vi "Process.vi"(8 "error in":errorcluster, 11 "RemoteControl":refnum<class "RemoteControl.lvclass">) -> (0 "error out":errorcluster, 3 "RemoteControl out":refnum<class "RemoteControl.lvclass">)   [LabVIEW 2020, in "RemoteControl.lvclass"]
doc: "---------------------------------------------------------------\nJKI State Machine Objects™\nhttp://jki.net/state-machine-objects/\nCopyright (C) 2005-2015, JKI <info@jki.net>\nALL RIGHTS RESERVED"
uses:
  RemoteControl.lvclass
  C:/Program Files (x86)/National Instruments/LabVIEW 2020/vi.lib/JKI/JKI SMO/SMO/SMO.lvclass
  Typedefs/RC Process Type--Enum.ctl
  Typedefs/Message--Cluster.ctl
  <vilib>/JKI/JKI SMO/SMO/Typedefs/Parent Call--Enum.ctl
  RemoteControl.lvclass/RemoteControl.ctl
  Typedefs/PublicEvents--RemoteControl.SendMessageFromProcess.ctl
  <vilib>/JKI/JKI SMO/SMO/Typedefs/SMOState --Enum.ctl
  LevyLab/LevyLab.lvclass
  <vilib>/JKI/JKI SMO/SMO/SMO.lvclass
panel:
  in  "Message Timing?":bool
  in  "timeout in ms (100)":i32=10
  out "Message from Remote":T1 {"Message ID" format="%#_6f"}
  out "Message from Owner":T1 {"Message ID" format="%#_6f"}
  in  "stop":bool
  out "RC Process Type":T2=enum."Server"
  # "For instructions on how to use the JKI State Machine Objects, examples and video tutorials, visit:\nhttp://jki.net/state-machine-objects/\n\nJKI State Machine Objects™\nhttp://jki.net/state-machine-objects/\nCopyright (C) 2005-2015, JKI <info@jki.net>\nALL RIGHTS RESERVED"
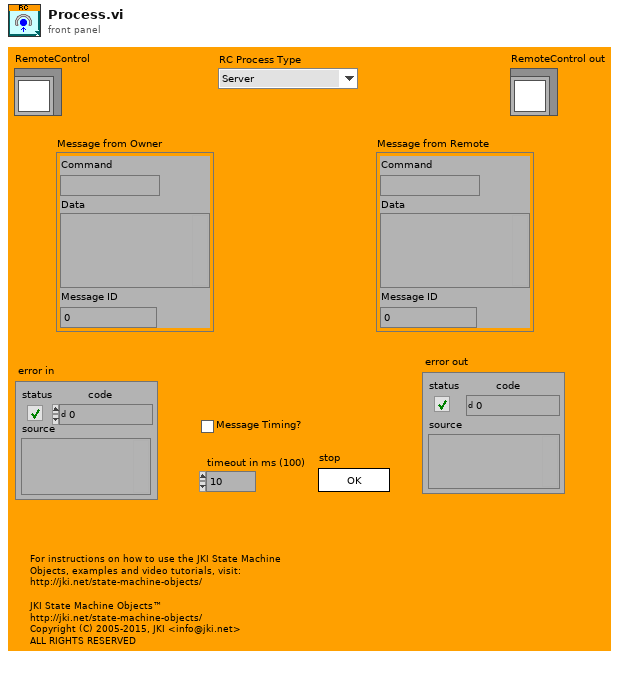
[diagram p1: front panel]
types:
  T1 = typedef "RemoteControl.lvclass/Message--Cluster.ctl" = cluster{"Command":string, "Data":variant, "Message ID":i32}
  T2 = typedef "RemoteControl.lvclass/RC Process Type--Enum.ctl" = enum16{"Connection Monitor", "Server", "Client"}
  T3 = typedef "SMO.lvclass/Parent Call--Enum.ctl" = enum16{"Allows parent to run", "Does not request parent to run"}
  T4 = enum32{"invalid app kind", "Development System", "Run Time System", "Student Edition", "Embedded LabVIEW", "Evaluation", "Custom"}
  T5 = enum32{"Invalid", "Standard", "Closed", "Hidden", "Minimized", "Maximized"}
  T6 = enum32{"Bad", "Idle", "Run top level", "Running"}
  T7 = typedef "RemoteControl.lvclass/PrivateEvents--RemoteControl.Configure.ctl" = cluster{"address":string, "Port":u16, "AllowedRemote":string, "Commands":string[], "Debug Mode?":bool}
  T8 = cluster{"Core":cluster{"Current VI Reference":refnum<vi>, "Close Panel on Exit?":bool, "error":errorcluster}, "Self Reference":refnum<class "RemoteControl.lvclass">, "RC Process Type":T2, "Configure":T7, "Message":T1, "Server":refnum<class "RemoteControl.lvclass">, "Debug Mode?":bool}
  T9 = cluster{"Current VI Reference":refnum<vi>, "Close Panel on Exit?":bool, "error":errorcluster}
  T10 = typedef "SMO.lvclass/Protected Events.ctl" = cluster{"StopProcesses":refnum<user-event>, "AbortProcesses":refnum<user-event>, "Config Changed":refnum<user-event>, "Dependency":refnum<user-event>}
  T11 = typedef "RemoteControl.lvclass/PrivateEvents--Cluster.ctl" = cluster{"Configure":refnum<user-event>, "SendMessageToProcess":refnum<user-event>}
  T12 = typedef "RemoteControl.lvclass/PublicEvents--Cluster.ctl" = cluster{"SendMessageFromProcess":refnum<user-event>}
  T13 = typedef "SMO.lvclass/Public Events.ctl" = cluster{"Error":refnum<user-event>, "State":refnum<user-event>, "Reserve State":refnum<user-event>}
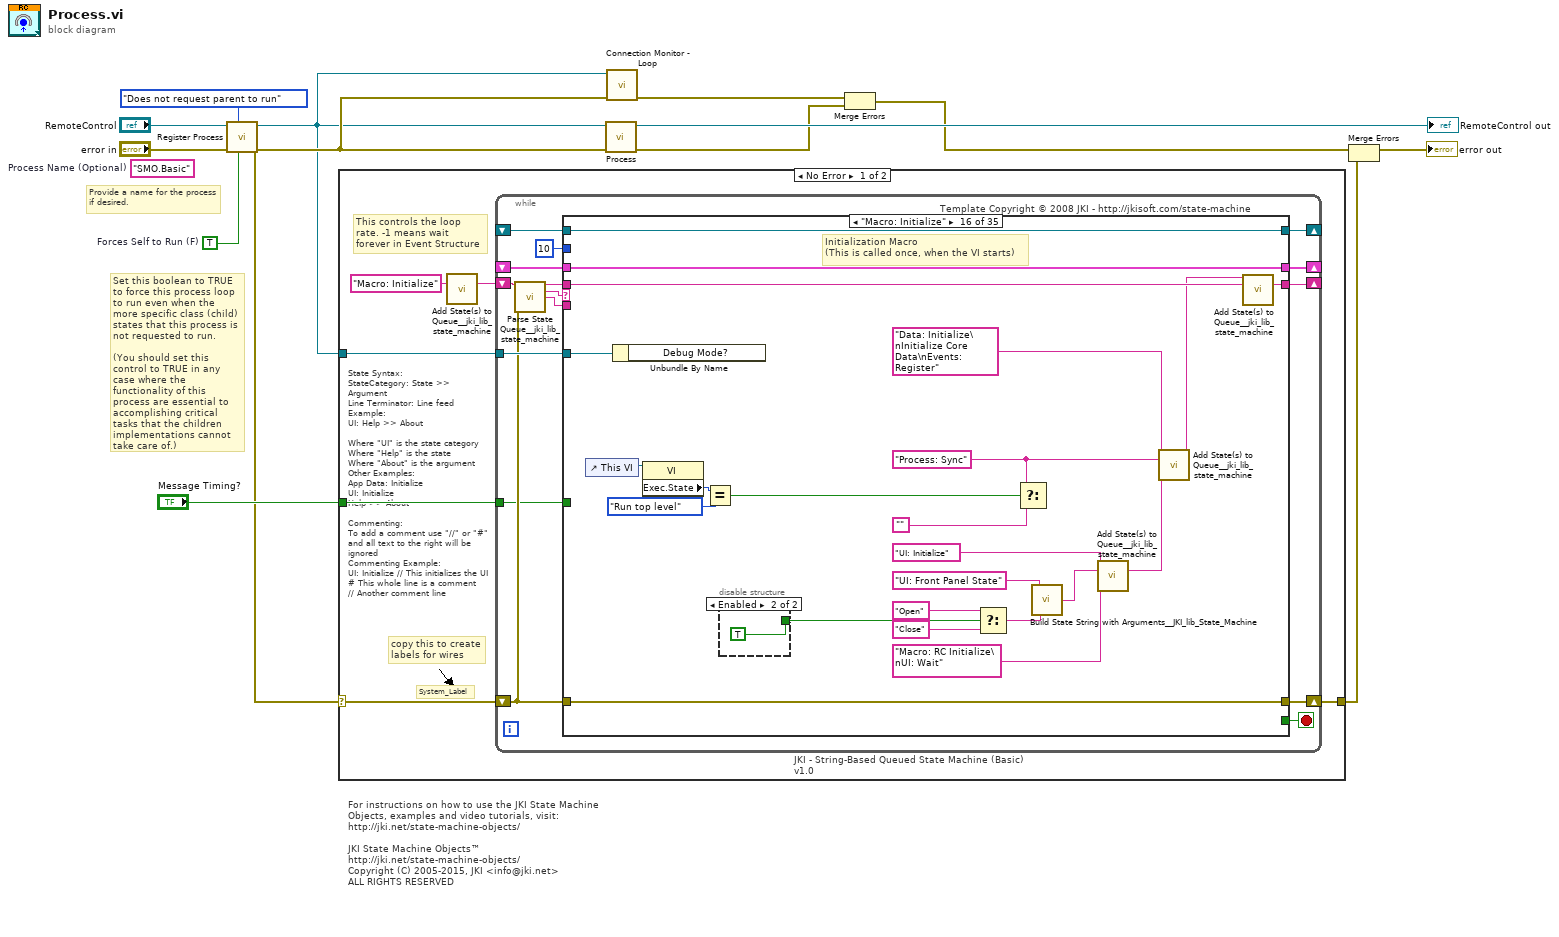
[diagram p0: block diagram]
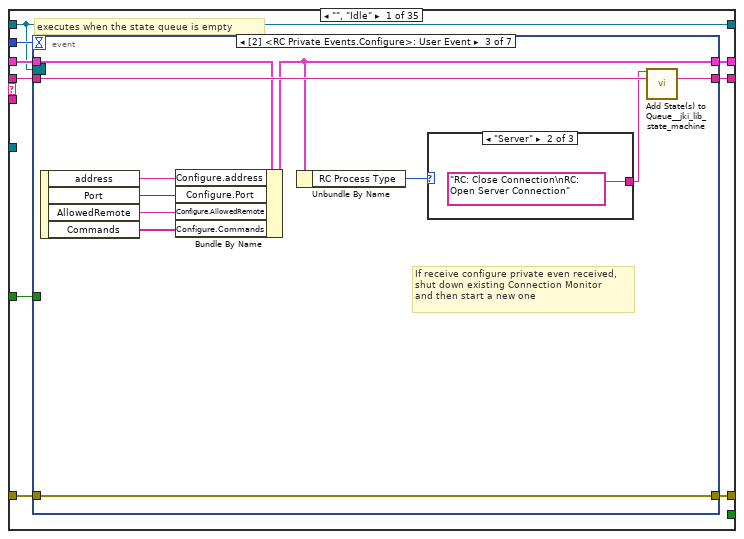
[diagram p2: hidden frame]
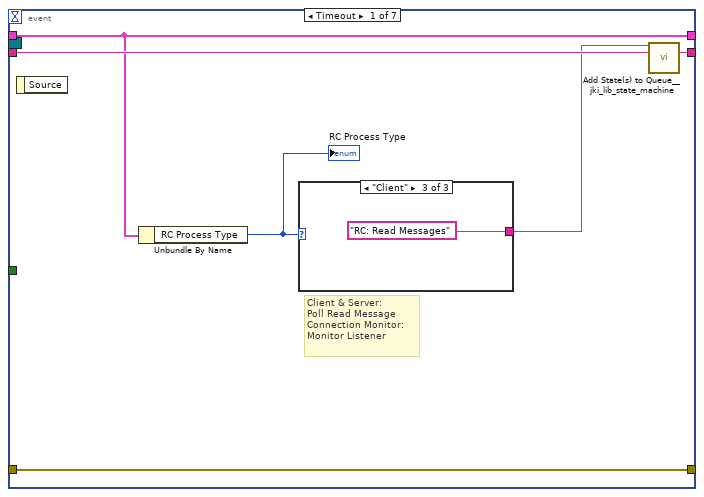
[diagram p3: hidden frame]
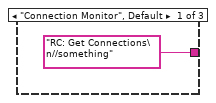
[diagram p4: hidden frame]
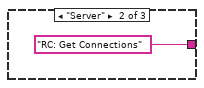
[diagram p5: hidden frame]
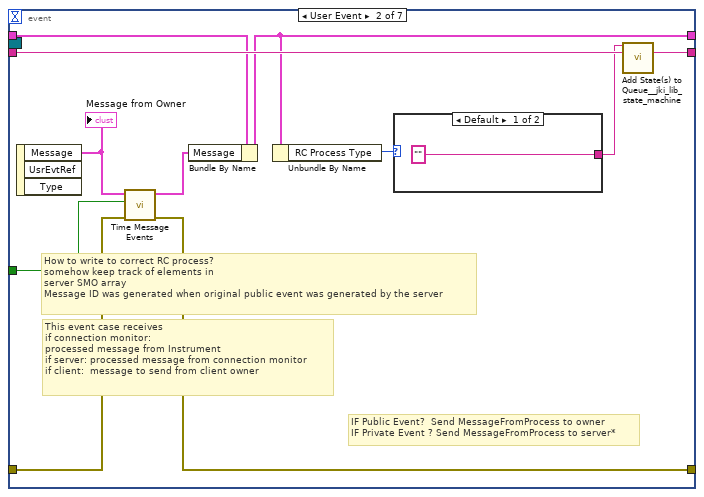
[diagram p6: hidden frame]
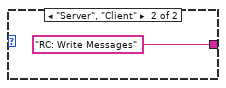
[diagram p7: hidden frame]
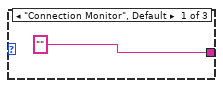
[diagram p8: hidden frame]
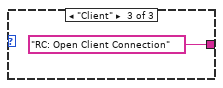
[diagram p9: hidden frame]
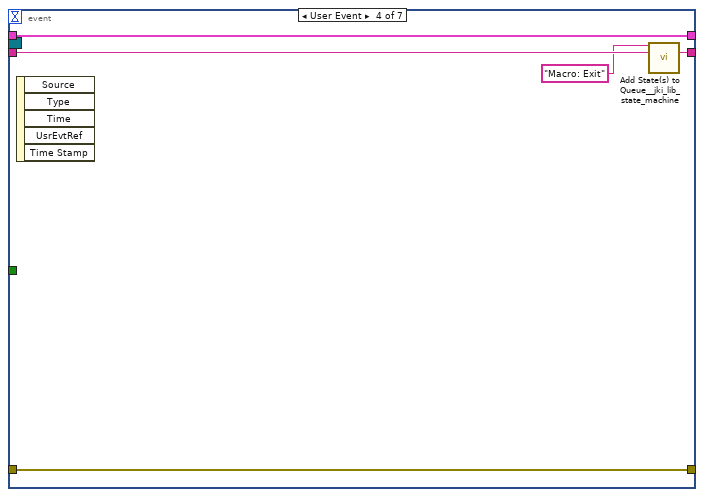
[diagram p10: hidden frame]
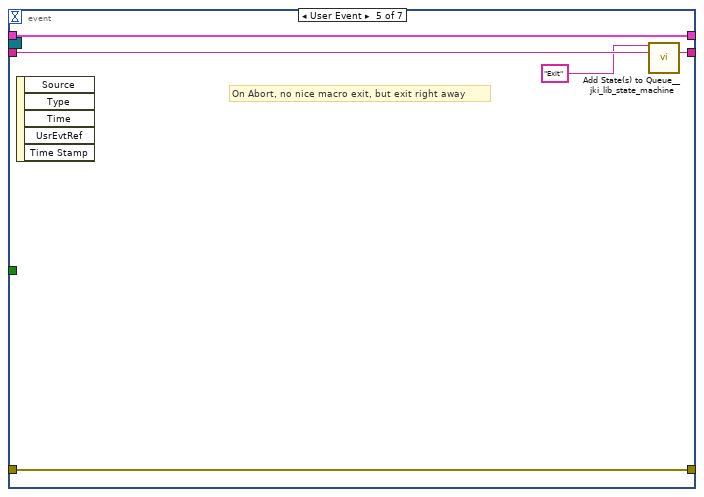
[diagram p11: hidden frame]
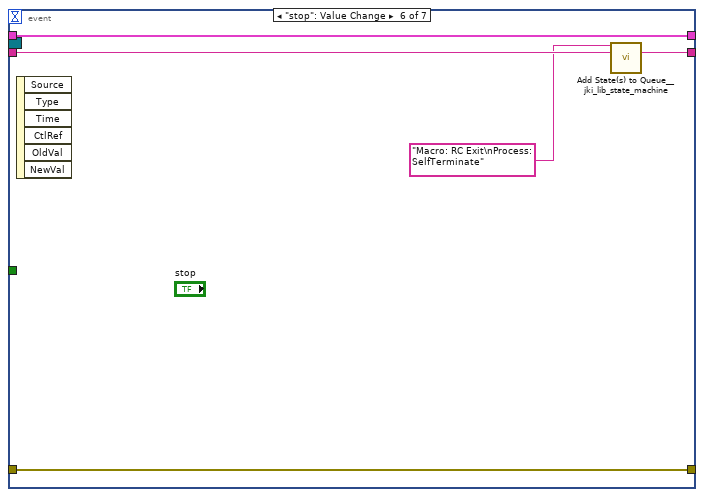
[diagram p12: hidden frame]
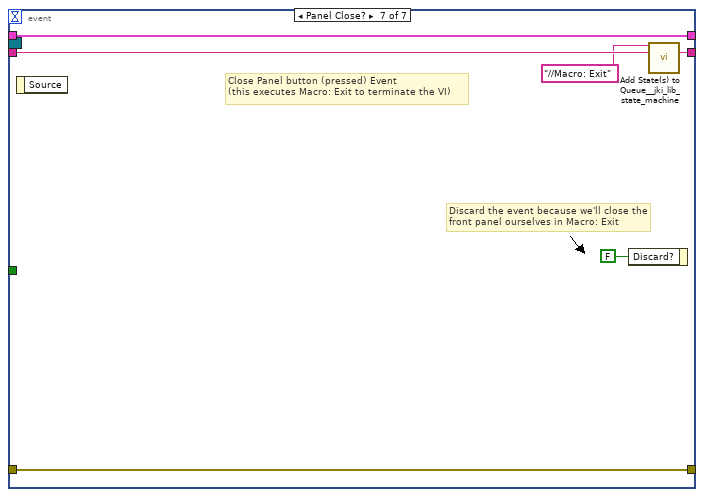
[diagram p13: hidden frame]
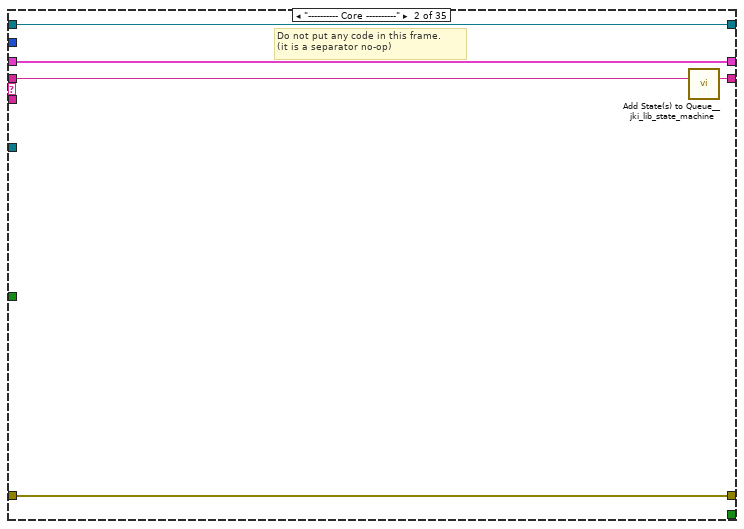
[diagram p14: hidden frame]
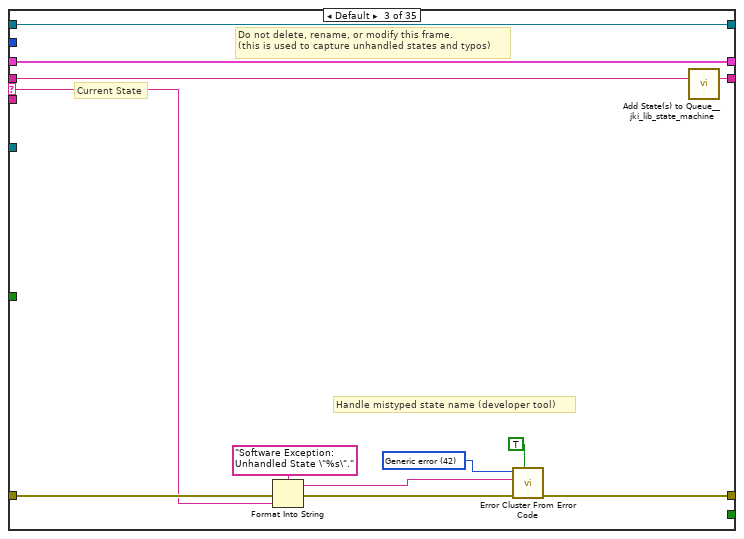
[diagram p15: hidden frame]
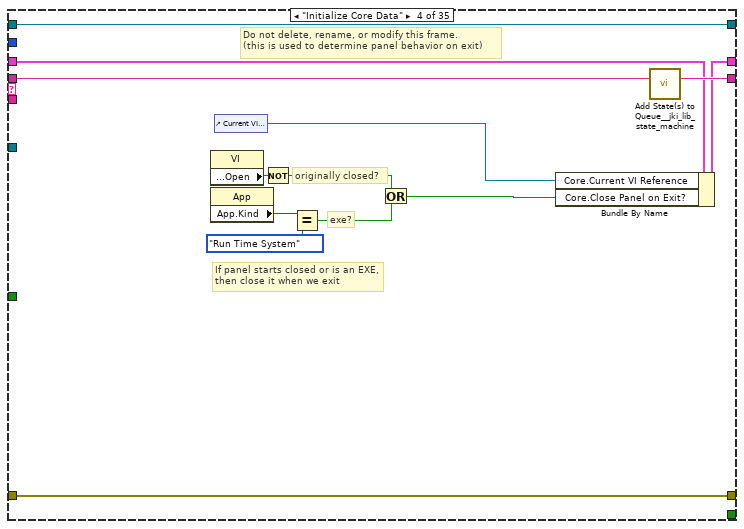
[diagram p16: hidden frame]
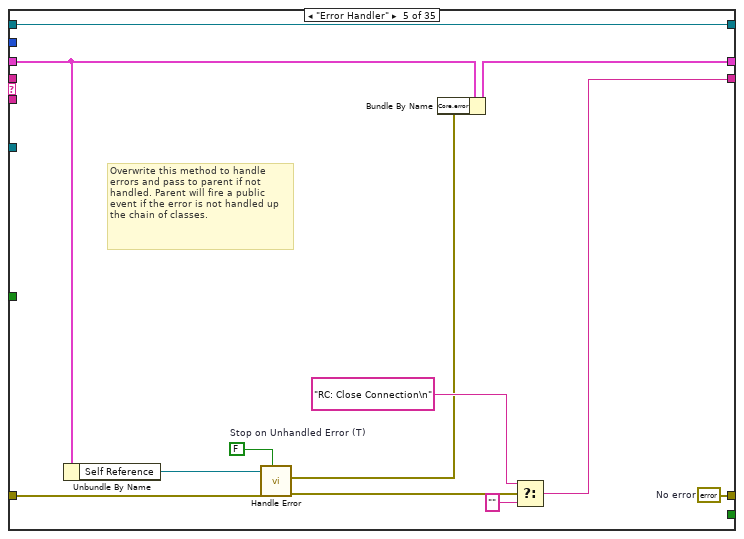
[diagram p17: hidden frame]
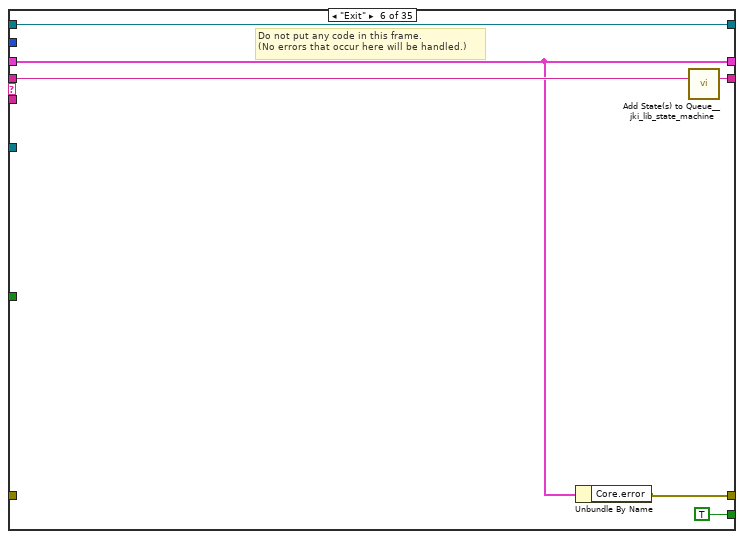
[diagram p18: hidden frame]
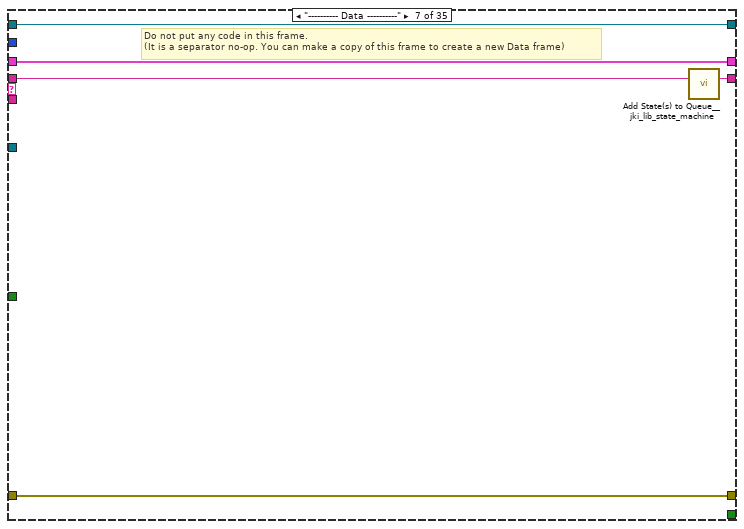
[diagram p19: hidden frame]
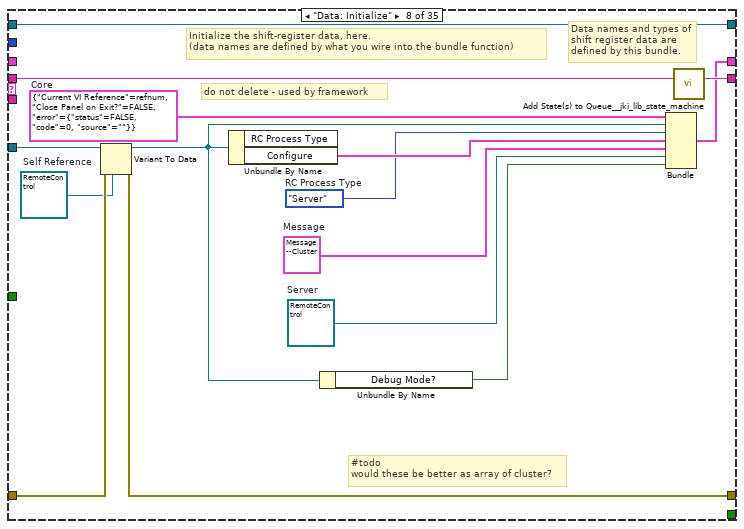
[diagram p20: hidden frame]
diagram:
  w7 = TRUE  # Forces Self to Run (F)
  (unwired) "SMO.Basic"  # Process Name (Optional)
  # "Provide a name for the process\nif desired."
  # "Set this boolean to TRUE to force this process loop to run even when the more specific class (child) states that this process is not requested to run.\n\n(You should set this control to TRUE in any case where the functionality of this process are essential to accomplishing critical tasks that the children implementations cannot take care of.)"
  # "For instructions on how to use the JKI State Machine Objects, examples and video tutorials, visit:\nhttp://jki.net/state-machine-objects/\n\nJKI State Machine Objects™\nhttp://jki.net/state-machine-objects/\nCopyright (C) 2005-2015, JKI <info@jki.net>\nALL RIGHTS RESERVED"
  n1 = call <vilib>:"Register Process.vi"("Forces Self to Run (F)"=w7, "Parent Call"=Parent_Call--Enum."Does not request parent to run", "error in (no error)"="error in", "SMO"="RemoteControl") -> ("error out"=w2:errorcluster, "SMO out"=w1:refnum<class "RemoteControl.lvclass">)  [unwired: 6 in]
  n2 = case shown="No Error" w2 {
    selector: w2 -> [w16 w489]
    tunnel: w1 -> [w17 _]
    tunnel: [w15 w489] -> w9
    tunnel: "Message Timing?" -> [w14 _]
    frame No Error {
      # "State Syntax:\nStateCategory: State >> Argument\nLine Terminator: Line feed\nExample:\nUI: Help >> About\n\nWhere \"UI\" is the state category\nWhere \"Help\" is the state\nWhere \"About\" is the argument\nOther Examples:\nApp Data: Initialize\nUI: Initialize\nHelp >> About\n\nCommenting:\nTo add a comment use \"//\" or \"#\" and all text to the right will be ignored\nCommenting Example:\nUI: Initialize // This initializes the UI\n# This whole line is a comment\n// Another comment line"
      # "copy this to create labels for wires"
      # "This controls the loop rate. -1 means wait forever in Event Structure"
      # "System_Label"
      n3 = call <vilib>:"Add State(s) to Queue__jki_lib_state_machine.vi"("State(s) in (\"\")"="Macro: Initialize") -> ("States Out"=w19:string)  [unwired: 14 in]
      n4 = while "JKI - String-Based Queued State Machine (Basic) v1.0" {
        shift-right: [w27] -> _
        shift-left: _ -> [w20]
        shift-right: [w30] -> w15
        shift-left: w16 -> [w22]
        shift-right: [w29] -> _
        shift-left: w19 -> [w31]
        tunnel: w17 -> [w25]
        shift-right: [w24] -> _
        shift-left: _ -> [w23]
        tunnel: w14 -> [w21]
        stop <- w28 stop-if-true
        # "Template Copyright © 2008 JKI - http://jkisoft.com/state-machine"
        n5 = call <vilib>:"Parse State Queue__jki_lib_state_machine.vi"("State Queue"=w31, "Error In (no error)"=w22) -> ("Remaining States"=w33:string, "Current State"=w34:string, "Arguments"=w32:string)  [unwired: 11 in]
        n6 = case shown="\"Macro: Initialize\"" w34 {
          selector: w34 -> [_ _ w107 _ _ _ _ _ _ _ _ _ _ _ _ _ _ _ _ _ _ _ _ _ _ _ _ _ _ _ _ _ _ _ _]
          tunnel: w33 -> [w43 w105 w111 w130 _ w148 w153 w168 w175 w180 w185 w192 w208 w243 w248 w271 w277 w291 w310 w315 w326 w335 w340 w359 w365 w370 w379 w391 w402 w421 w450 w459 w466 w475 w488]
          tunnel: w32 -> [_ _ _ _ _ _ _ _ _ _ _ w186 w203 _ _ _ _ _ _ _ _ _ _ _ _ _ _ _ _ _ _ _ _ _ _]
          tunnel: [w40 w103 w113 w127 w141 w143 w151 w165 w172 w178 w181 w187 w201 w234 w246 w269 w278 w289 w308 w313 w318 w327 w338 w353 w361 w366 w376 w387 w396 w409 w446 w451 w460 w470 w485] -> w30
          tunnel: w22 -> [w39 w103 w112 w127 w136 _ w151 w166 w173 w178 w181 w188 w206 w235 w246 w269 w278 w289 w308 w313 w319 w328 w338 w354 w361 w366 w375 w382 w397 w418 w442 w452 w461 w471 w478]
          tunnel: [w42 w104 w110 w129 w131 w147 w152 w167 w174 w179 w184 w191 w207 w242 w247 w270 w282 w290 w309 w314 w325 w334 w339 w358 w364 w369 w378 w390 w401 w420 w449 w458 w465 w474 w487] -> w29
          tunnel: [_ _ _ _ _ TRUE _ _ _ _ _ _ _ _ _ _ _ _ _ _ _ _ _ _ _ _ _ _ _ _ _ _ _ _ _] -> w28
          tunnel: [w38 w102 w109 w128 w139 w144 w150 w160 w171 w177 w182 w190 w205 w238 w245 w267 w279 w286 w303 w312 w323 w332 w337 w357 w363 w368 w373 w388 w394 w407 w445 w454 w463 w467 w484] -> w27
          tunnel: 10 ("Timeout") -> [w37 _ _ _ _ _ _ _ _ _ _ _ _ _ _ _ _ _ _ _ _ _ _ _ _ _ _ _ _ _ _ _ _ _ _]
          tunnel: w25 -> [_ _ _ _ _ _ _ w163 _ _ _ _ _ _ _ w258 _ _ _ _ _ _ _ _ _ _ _ _ _ _ _ _ _ _ _]
          tunnel: [w36 w101 w106 w118 w142 w145 w149 w162 w170 w176 w183 w189 w202 w241 w244 w268 w281 w288 w304 w311 w324 w333 w336 w356 w362 w367 w377 w389 w400 w419 w448 w457 w464 w473 w486] -> w24
          tunnel: w23 -> [w36 w101 w106 w118 w142 w145 w149 w162 w170 w176 w183 w189 w202 w241 w244 w268 w281 w288 w304 w311 w324 w333 w336 _ w362 w367 w377 w389 w400 w419 w448 w457 w464 w473 w486]
          tunnel: w21 -> [w35 _ _ _ _ _ _ _ _ _ _ _ _ _ _ _ _ _ _ _ _ _ _ _ _ _ _ w383 _ w406 w444 _ _ _ _]
          tunnel: w20 -> [w41 w102 w109 w121 w140 w144 w150 _ w171 w177 w182 w190 w205 w238 w245 w267 w279 w286 w303 w312 w323 w331 w337 w357 w363 w368 w372 w388 w393 w408 w445 w455 w463 w468 w483]
          frame "", "Idle" {
            # "executes when the state queue is empty"
            n7 = event shown="[2] <RC Private Events.Configure>: User Event" {
              selector: w36 -> [_ _ _ _ _ _ _]
              dyn-events: _ -> [_ _ _ _ _ _ _]
              timeout: w37 -> [_ _ _ _ _ _ _]
              tunnel: w43 -> [w49 w63 w75 w84 w89 w93 w100]
              tunnel: [w48 w62 w74 w83 w88 w94 w99] -> w42
              tunnel: w41 -> [w45 w61 w73 w81 w86 w92 w97]
              tunnel: [w47 w54 w76 w82 w87 w90 w98] -> w40
              tunnel: w39 -> [w47 w55 w76 w82 w87 w90 w98]
              tunnel: [w45 w59 w71 w81 w86 w92 w97] -> w38
              tunnel: w35 -> [_ w53 _ _ _ _ _]
              event Timeout {
                # "Client & Server:\nPoll Read Message\nConnection Monitor:\nMonitor Listener"
                n8 = event-data() -> ()  [unwired: 1 in, 1 out]
                n9 = Unbundle By Name(w45) -> ("RC Process Type"=w44:T2)
                "RC Process Type" <- w44
                n10 = case shown="\"Client\"" w44 {
                  tunnel: ["RC: Get Connections\n//something" ("State(s) in Front (\"\")") "RC: Get Connections" ("State(s) in Front (\"\")") "RC: Read Messages" ("State(s) in Front (\"\")")] -> w46
                  frame "Connection Monitor", Default {
                  }
                  frame "Server" {
                  }
                  frame "Client" {
                  }
                }
                n11 = call <vilib>:"Add State(s) to Queue__jki_lib_state_machine.vi"("State(s) in Front (\"\")"=w46, "State(s) in (\"\")"=w49) -> ("States Out"=w48:string)  [unwired: 13 in]
              }
              event User Event {
                # "IF Public Event?  Send MessageFromProcess to owner\nIF Private Event ? Send MessageFromProcess to server*"
                # "How to write to correct RC process?\nsomehow keep track of elements in\nserver SMO array\nMessage ID was generated when original public event was generated by the server"
                # "This event case receives\nif connection monitor:\nprocessed message from Instrument\nif server: processed message from connection monitor\nif client:  message to send from client owner"
                n12 = event-data() -> ("Message"=w57:T1)  [unwired: 1 in, 2 out]
                "Message from Owner" <- w57
                n13 = call "Time Message Events.vi"("error in (no error)"=w55, "Debug Mode"=w53, "Message in"=w57) -> ("error out"=w54:errorcluster, "Message out"=w56:T1)  [unwired: 6 in, 1 out]
                n14 = Bundle By Name(cluster=w61, "Message"=w56) -> (w59:T8)
                n15 = Unbundle By Name(w59) -> ("RC Process Type"=w60:T2)
                n16 = case shown="Default" w60 {
                  tunnel: ["" ("State(s) in Front (\"\")") "RC: Write Messages" ("State(s) in Front (\"\")")] -> w58
                  frame Default {
                  }
                  frame "Server", "Client" {
                  }
                }
                n17 = call <vilib>:"Add State(s) to Queue__jki_lib_state_machine.vi"("State(s) in Front (\"\")"=w58, "State(s) in (\"\")"=w63) -> ("States Out"=w62:string)  [unwired: 13 in]
              }
              event User Event {
                # "If receive configure private even received,\nshut down existing Connection Monitor \nand then start a new one"
                n18 = event-data() -> ("address"=w66:string, "Port"=w67:u16, "AllowedRemote"=w68:string, "Commands"=w69:string[])  [unwired: 1 in]
                n19 = Bundle By Name(cluster=w73, "Configure.address"=w66, "Configure.Port"=w67, "Configure.AllowedRemote"=w68, "Configure.Commands"=w69) -> (w71:T8)
                n20 = Unbundle By Name(w71) -> ("RC Process Type"=w72:T2)
                n21 = case shown="\"Server\"" w72 {
                  tunnel: ["" ("State(s) in Front (\"\")") "RC: Close Connection\nRC: Open Server Connection" "RC: Open Client Connection"] -> w70
                  frame "Connection Monitor", Default {
                  }
                  frame "Server" {
                  }
                  frame "Client" {
                  }
                }
                n22 = call <vilib>:"Add State(s) to Queue__jki_lib_state_machine.vi"("State(s) in Front (\"\")"=w70, "State(s) in (\"\")"=w75) -> ("States Out"=w74:string)  [unwired: 13 in]
              }
              event User Event {
                n23 = event-data() -> ()  [unwired: 1 in, 5 out]
                n24 = call <vilib>:"Add State(s) to Queue__jki_lib_state_machine.vi"("State(s) in Front (\"\")"="Macro: Exit", "State(s) in (\"\")"=w84) -> ("States Out"=w83:string)  [unwired: 13 in]
              }
              event User Event {
                # "On Abort, no nice macro exit, but exit right away"
                n25 = event-data() -> ()  [unwired: 1 in, 5 out]
                n26 = call <vilib>:"Add State(s) to Queue__jki_lib_state_machine.vi"("State(s) in Front (\"\")"="Exit", "State(s) in (\"\")"=w89) -> ("States Out"=w88:string)  [unwired: 13 in]
              }
              event "stop": Value Change {
                n27 = event-data() -> ()  [unwired: 1 in, 6 out]
                n28 = call <vilib>:"Add State(s) to Queue__jki_lib_state_machine.vi"("State(s) in Front (\"\")"="Macro: RC Exit\nProcess: SelfTerminate" ("State(s) in Front (\"\")"), "State(s) in (\"\")"=w93) -> ("States Out"=w94:string)  [unwired: 13 in]
              }
              event Panel Close? {
                # "Discard the event because we'll close the front panel ourselves in Macro: Exit"
                # "Close Panel button (pressed) Event\n(this executes Macro: Exit to terminate the VI)"
                n29 = event-data() -> ()  [unwired: 1 in, 1 out]
                n30 = event-data("Discard?"=FALSE) -> ()  [unwired: 1 in, 1 out]
                n31 = call <vilib>:"Add State(s) to Queue__jki_lib_state_machine.vi"("State(s) in Front (\"\")"="//Macro: Exit", "State(s) in (\"\")"=w100) -> ("States Out"=w99:string)  [unwired: 13 in]
              }
            }
          }
          frame "---------- Core ----------" {
            # "Do not put any code in this frame.\n(it is a separator no-op)"
            n32 = call <vilib>:"Add State(s) to Queue__jki_lib_state_machine.vi"("State(s) in (\"\")"=w105) -> ("States Out"=w104:string)  [unwired: 14 in]
          }
          frame Default {
            w116 = 42 items=["No error", "Argument error", "Memory is full", "Out of zone", "End of file", "File already open", "Generic file I/O error", "File not found", "File permission error", "Disk is full", "Duplicate path", "Too many files open", "System feature not enabled", "Resource file not found", "Cannot add resource", "Resource not found", "Image not found", "Image memory error", "Pen does not exist", "Config type invalid", "Config token not found", "Config parse error", "Config memory error", "Bad external code format", "Bad external code offset", "External code not present", "Null window", "Destroy window error", "Null menu", "Print aborted", "Bad print record", "Print driver error", "Windows error during printing", "Memory error during printing", "Print dialog error", "Generic print error", "Invalid device refnum", "Device not found", "Device parameter error", "Device unit error", "Cannot open device", "Device call aborted", "Generic error", "Cancelled by user", "Object ID too low", "Object ID too high", "Object not in heap", "Unknown heap", "Unknown object (invalid DefProc)", "Unknown object (DefProc not in table)", "Message out of range", "Invalid (null) method", "Unknown message", "Manager call not supported", "Bad address", "Network operation in progress", "Network operation timed out", "Connection is busy", "Network attribute not supported", "Network error", "Address in use", "System out of memory", "Connection aborted", "Connection refused", "Not connected", "Already connected", "Connection closed", "Initialization error (interapplication manager)", "Bad occurrence", "Wait on unbound occurrence handler", "Occurrence queue overflow", "Datalog type conflict", "Unused", "Unrecognized type (interapplication manager)", "Memory corrupt", "Failed to make temporary DLL", "Old CIN version", "Drag socket not found", "Failed to load drop-object", "Failed to register OLE object", "Failed to release OLE object", "Format specifier type mismatch", "Unknown format specifier", "Too few format specifiers", "Too many format specifiers", "Scan failed", "Newer CIN version", "Error converting to variant", "Runtime menu error", "Password tampered", "Variant attribute not found", "Incompatible variant data type", "Event data is not available", "Event Store is not present", "Occurrence is not found", "Event Queue is not created", "Event info is not available", "Refnum passed is NULL", "Error retrieving Class GUID", "Error retrieving CoClass GUID", "Error retrieving TypeLib GUID.", "Bad built application magic bytes.", "Specific driver is different from the specific driver associated with the Logical Name.", "There is no session opened to the class driver.", "Max Error", "MAX - Error with config objects", "MAX - Error loading configuration", "MAX - Group not supported"]
            # "Current State"
            # "Do not delete, rename, or modify this frame.\n(this is used to capture unhandled states and typos)"
            # "Handle mistyped state name (developer tool)"
            n33 = Format Into String(format string="Software Exception: Unhandled State \"%s\"." ("message"), error in=w112, w107) -> (resulting string=w115:string, error out=w114:errorcluster)  [unwired: 1 in]
            n34 = call <vilib>:"Error Cluster From Error Code.vi"("show call chain? (False)"=TRUE, "error in (no error)"=w114, "error message (\"\")"=w115, "error code (0)"=w116) -> ("error out"=w113:errorcluster)  [unwired: 5 in]
            n35 = call <vilib>:"Add State(s) to Queue__jki_lib_state_machine.vi"("State(s) in (\"\")"=w111) -> ("States Out"=w110:string)  [unwired: 14 in]
          }
          frame "Initialize Core Data" {
            # "Do not delete, rename, or modify this frame.\n(this is used to determine panel behavior on exit)"
            # "originally closed?"
            # "exe?"
            # "If panel starts closed or is an EXE, then close it when we exit"
            n36 = property class="VI"() -> ("Front Panel.Open"=w126:bool)  [unwired: 2 in, 2 out]
            n37 = property class="App"() -> ("App.Kind"=w125:T4)  [unwired: 2 in, 2 out]
            n38 = control-ref of="Current VI Reference"() -> (w119:refnum<vi>)
            n39 = Not(x=w126) -> (.not. x?=w123:bool)
            n40 = Equal?(x=w125, y=T4."Run Time System" ("Application:Kind")) -> (x = y?=w122:bool)
            n41 = Or(x=w123, y=w122) -> (x .or. y?=w120:bool)
            n42 = Bundle By Name(cluster=w121, "Core.Current VI Reference"=w119, "Core.Close Panel on Exit?"=w120) -> (w128:T8)
            n43 = call <vilib>:"Add State(s) to Queue__jki_lib_state_machine.vi"("State(s) in (\"\")"=w130) -> ("States Out"=w129:string)  [unwired: 14 in]
          }
          frame "Error Handler" {
            w137 = FALSE  # Stop on Unhandled Error (T)
            w141 = errorcluster {"status"=FALSE, "code"=0, "source"=""}  # No error
            # "Overwrite this method to handle errors and pass to parent if not handled. Parent will fire a public event if the error is not handled up the chain of classes."
            n44 = Unbundle By Name(w140) -> ("Self Reference"=w135:refnum<class "RemoteControl.lvclass">)
            n45 = call-dynamic "Handle Error.vi"("Stop on Unhandled Error (T)"=w137, "error in"=w136, "LevyLab"=w135) -> ("handling error"=w133:errorcluster, "Unhandled error"=w134:errorcluster)  [unwired: 6 in, 1 out]
            n46 = Bundle By Name(cluster=w140, "Core.error"=w134) -> (w139:T8)
            n47 = Select(t="RC: Close Connection\n", s=w133, f="") -> (s? t:f=w131:string)
          }
          frame "Exit" {
            # "Do not put any code in this frame.\n(No errors that occur here will be handled.)"
            n48 = Unbundle By Name(w144) -> ("Core.error"=w143:errorcluster)
            n49 = call <vilib>:"Add State(s) to Queue__jki_lib_state_machine.vi"("State(s) in (\"\")"=w148) -> ("States Out"=w147:string)  [unwired: 14 in]
          }
          frame "---------- Data ----------" {
            # "Do not put any code in this frame.\n(It is a separator no-op. You can make a copy of this frame to create a new Data frame)"
            n50 = call <vilib>:"Add State(s) to Queue__jki_lib_state_machine.vi"("State(s) in (\"\")"=w153) -> ("States Out"=w152:string)  [unwired: 14 in]
          }
          frame "Data: Initialize" {
            w156 = RC_Process_Type--Enum."Server"  # RC Process Type
            w157 = refnum<class "RemoteControl.lvclass"> refnum  # Server
            w158 = T1 {"Command"="", "Data"=variant, "Message ID"=0}  # Message
            w161 = T9 {"Current VI Reference"=refnum, "Close Panel on Exit?"=FALSE, "error"={"status"=FALSE, "code"=0, "source"=""}}  # Core
            w164 = refnum<class "RemoteControl.lvclass"> refnum  # Self Reference
            # "#todo\nwould these be better as array of cluster?"
            # "do not delete - used by framework"
            # "Data names and types of shift register data are defined by this bundle."
            # "Initialize the shift-register data, here.\n(data names are defined by what you wire into the bundle function)"
            n51 = Variant To Data(error in=w166, type=w164, Variant=w163) -> (data=w155:refnum<class "RemoteControl.lvclass">, error out=w165:errorcluster)
            n52 = Unbundle By Name(w155) -> ("Configure"=w159:T7)  [unwired: 1 out]
            n53 = Unbundle By Name(w155) -> ("Debug Mode?"=w154:bool)
            n54 = Bundle("Core"=w161, "Self Reference"=w155, "RC Process Type"=w156, "Configure"=w159, "Message"=w158, "Server"=w157, "Debug Mode?"=w154) -> (w160:T8)  [unwired: 1 in]
            n55 = call <vilib>:"Add State(s) to Queue__jki_lib_state_machine.vi"("State(s) in (\"\")"=w168) -> ("States Out"=w167:string)  [unwired: 14 in]
          }
          frame "Data: Cleanup" {
            # "Cleanup any data and references, here.\n(this is called automatically, by the Macro: Exit)"
            n56 = Unbundle By Name(w171) -> ("Core.Current VI Reference"=w169:refnum<vi>)
            n57 = Close Reference(reference=w169, error in (no error)=w173) -> (error out=w172:errorcluster)
            n58 = call <vilib>:"Add State(s) to Queue__jki_lib_state_machine.vi"("State(s) in (\"\")"=w175) -> ("States Out"=w174:string)  [unwired: 14 in]
          }
          frame "---------- UI ----------" {
            # "Do not put any code in this frame.\n(It is a separator no-op. You can make a copy of this frame to create a new UI frame)"
            n59 = call <vilib>:"Add State(s) to Queue__jki_lib_state_machine.vi"("State(s) in (\"\")"=w180) -> ("States Out"=w179:string)  [unwired: 14 in]
          }
          frame "UI: Initialize" {
            # "Initialize the User Interface, here.\n(this is called automatically, by the Macro: Init)"
            n60 = call <vilib>:"Add State(s) to Queue__jki_lib_state_machine.vi"("State(s) in (\"\")"=w185) -> ("States Out"=w184:string)  [unwired: 14 in]
          }
          frame "UI: Cursor Set" {
            # "Argument"
            # "Initialize the User Interface, here.\n(this is called automatically, by the Macro: Init)"
            n61 = disable-structure shown="Default" {
              disable-tunnel: w188 -> [w193 w196]
              disable-tunnel: [w193 w195] -> w187
              disable-tunnel: w186 -> [_ w194]
              frame condition #0 {
              }
              frame condition #1 (active) {
                n62 = case shown="\"Idle\", Default" w194 {
                  tunnel: w196 -> [w198 w200]
                  tunnel: [w197 w199] -> w195
                  frame "Idle", Default {
                    n63 = call <vilib>:"Unset Busy.vi"("error in (no error)"=w198) -> ("error out"=w197:errorcluster)  [unwired: 10 in]
                  }
                  frame "Busy" {
                    n64 = call <vilib>:"Set Busy.vi"("error in (no error)"=w200) -> ("error out"=w199:errorcluster)  [unwired: 9 in, 1 out]
                  }
                }
              }
            }
            n65 = call <vilib>:"Add State(s) to Queue__jki_lib_state_machine.vi"("State(s) in (\"\")"=w192) -> ("States Out"=w191:string)  [unwired: 14 in]
          }
          frame "UI: Front Panel State" {
            # "Argument"
            # "Set Front Panel Open or Closed\n(Usage: \"UI: Front Panel State >> Open|Close\")"
            n66 = Unbundle By Name(w205) -> ("Core.Current VI Reference"=w204:refnum<vi>)
            n67 = disable-structure shown="Default" {
              disable-tunnel: w206 -> [w212 w233]
              disable-tunnel: [w211 w233] -> w201
              disable-tunnel: w204 -> [w210 _]
              disable-tunnel: w203 -> [w209 _]
              frame condition #0 (active) {
                n68 = case shown="\"Close\"" w209 {
                  tunnel: w212 -> [w216 w227]
                  tunnel: [w217 w228] -> w211
                  tunnel: w210 -> [_ _]
                  frame "Open", Default {
                    n69 = property class="VI"(error in=w216) -> (reference out=w214:refnum<vi>, error out=w215:errorcluster, "FP.State"=w213:T5)  [unwired: 1 in]
                    n70 = case shown="\"Closed\"" w213 {
                      tunnel: [w220 w223] -> w217
                      tunnel: w215 -> [w219 w223]
                      tunnel: w214 -> [w218 _]
                      frame "Closed" {
                        n71 = invoke class="VI" method="FP.Open"(reference=w218, error in=w219, "Activate"=TRUE, "State"=T5."Standard") -> (error out=w220:errorcluster)  [unwired: 1 in, 4 out]
                      }
                      frame Default {
                      }
                    }
                  }
                  frame "Close" {
                    n72 = property class="VI"(error in=w227) -> (reference out=w225:refnum<vi>, error out=w226:errorcluster, "FP.State"=w224:T5)  [unwired: 1 in]
                    n73 = case shown="Default" w224 {
                      tunnel: [w229 w232] -> w228
                      tunnel: w226 -> [w229 w231]
                      tunnel: w225 -> [_ w230]
                      frame "Invalid", "Closed" {
                      }
                      frame Default {
                        n74 = invoke class="VI" method="FP.Close"(reference=w230, error in=w231) -> (error out=w232:errorcluster)  [unwired: 1 in, 2 out]
                      }
                    }
                  }
                }
              }
              frame condition #1 {
              }
            }
            n75 = call <vilib>:"Add State(s) to Queue__jki_lib_state_machine.vi"("State(s) in (\"\")"=w208) -> ("States Out"=w207:string)  [unwired: 14 in]
          }
          frame "UI: Wait" {
            # "Do not put any code in this frame.\n(It is a separator no-op. You can make a copy of this frame to create a new UI frame)"
            n76 = Unbundle By Name(w238) -> ("Debug Mode?"=w237:bool)
            n77 = Select(t=u32 5000, s=w237, f=u32 0 ("milliseconds to wait")) -> (s? t:f=w236:u32)
            n78 = call <userlib>:"Wait (ms)__ogtk.vi"("error in (no error)"=w235, "milliseconds to wait"=w236) -> ("error out"=w234:errorcluster)  [unwired: 8 in, 1 out]
            n79 = call <vilib>:"Add State(s) to Queue__jki_lib_state_machine.vi"("State(s) in (\"\")"=w243) -> ("States Out"=w242:string)  [unwired: 14 in]
          }
          frame "---------- Macro ----------" {
            # "Do not put any code in this frame.\n(It is a separator no-op. You can make a copy of this frame to create a new Macro frame)"
            n80 = call <vilib>:"Add State(s) to Queue__jki_lib_state_machine.vi"("State(s) in (\"\")"=w248) -> ("States Out"=w247:string)  [unwired: 14 in]
          }
          frame "Macro: Initialize" {
            w259 = "Process: Sync"
            # "Initialization Macro\n(This is called once, when the VI starts)"
            n81 = control-ref of="This VI"() -> (w261:refnum<vi>)
            n82 = Unbundle By Name(w258) -> ()  [unwired: 1 out]
            n83 = property class="VI"(reference=w261) -> ("Exec.State"=w260:T6)  [unwired: 1 in, 2 out]
            n84 = Equal?(x=w260, y=T6."Run top level") -> (x = y?=w265:bool)
            n85 = disable-structure shown="Enabled" {
              disable-tunnel: [TRUE TRUE] -> w249
              frame Disabled {
              }
              frame Enabled {
              }
            }
            n86 = Select(t="Open", s=w249, f="Close") -> (s? t:f=w255:string)
            n87 = Select(t=w259, s=w265, f="") -> ()  [unwired: 1 out]
            n88 = call <vilib>:"Build State String with Arguments__JKI_lib_State_Machine.vi"("Arguments (\"\")"=w255, "State"="UI: Front Panel State") -> ("State with Arguments"=w252:string)  [unwired: 4 in]
            n89 = call <vilib>:"Add State(s) to Queue__jki_lib_state_machine.vi"("State(s) in Front (\"\")"="UI: Initialize", "State(s) in (\"\")"=w252, "State(s) at Back (\"\")"="Macro: RC Initialize\nUI: Wait") -> ("States Out"=w250:string)  [unwired: 12 in]
            n90 = call <vilib>:"Add State(s) to Queue__jki_lib_state_machine.vi"("State(s) in Front (\"\")"="Data: Initialize\nInitialize Core Data\nEvents: Register", "State(s) in (\"\")"=w259, "State(s) at Back (\"\")"=w250) -> ("States Out"=w262:string)  [unwired: 12 in]
            n91 = call <vilib>:"Add State(s) to Queue__jki_lib_state_machine.vi"("State(s) in Front (\"\")"=w262, "State(s) in (\"\")"=w271) -> ("States Out"=w270:string)  [unwired: 13 in]
          }
          frame "Macro: RC Initialize" {
            n92 = Unbundle By Name(w279) -> ("RC Process Type"=w280:T2)
            n93 = case shown="\"Server\"" w280 {
              tunnel: ["" ("State(s) in Front (\"\")") "RC: Open Server Connection" ("State(s) in Front (\"\")") "RC: Open Client Connection" ("State(s) in Front (\"\")")] -> w275
              frame "Connection Monitor", Default {
              }
              frame "Server" {
              }
              frame "Client" {
              }
            }
            n94 = call <vilib>:"Add State(s) to Queue__jki_lib_state_machine.vi"("State(s) in Front (\"\")"="RC: Open Context", "State(s) in (\"\")"=w275) -> ("States Out"=w274:string)  [unwired: 13 in]
            n95 = call <vilib>:"Add State(s) to Queue__jki_lib_state_machine.vi"("State(s) in Front (\"\")"=w274, "State(s) in (\"\")"=w277) -> ("States Out"=w282:string)  [unwired: 13 in]
          }
          frame "Macro: RC Exit" {
            n96 = call <vilib>:"Add State(s) to Queue__jki_lib_state_machine.vi"("State(s) in Front (\"\")"="RC: Close Connection\nRC: Stop Listener" ("State(s) in Front (\"\")"), "State(s) in (\"\")"=w291) -> ("States Out"=w290:string)  [unwired: 13 in]
          }
          frame "Macro: Exit" {
            # "Exit Macro\n(This is called once, when the VI exits)"
            n97 = Unbundle By Name(w303) -> ("Debug Mode?"=w292:bool, "Core.Close Panel on Exit?"=w298:bool)
            n98 = Select(t="Open", s=w292, f="Close") -> (s? t:f=w295:string)
            n99 = call <vilib>:"Build State String with Arguments__JKI_lib_State_Machine.vi"("Arguments (\"\")"=w295, "State"="UI: Front Panel State") -> ("State with Arguments"=w293:string)  [unwired: 4 in]
            n100 = Select(t=w293, s=w298, f="") -> (s? t:f=w306:string)
            n101 = call <vilib>:"Add State(s) to Queue__jki_lib_state_machine.vi"("State(s) in Front (\"\")"="Macro: RC Exit\nData: Cleanup\nEvents: Unregister", "State(s) in (\"\")"="Process: Sync", "State(s) at Back (\"\")"="Exit") -> ("States Out"=w300:string)  [unwired: 12 in]
            n102 = call <vilib>:"Add State(s) to Queue__jki_lib_state_machine.vi"("State(s) in (\"\")"=w306, "State(s) at Back (\"\")"=w300) -> ("States Out"=w305:string)  [unwired: 13 in]
            n103 = call <vilib>:"Add State(s) to Queue__jki_lib_state_machine.vi"("State(s) in Front (\"\")"=w305, "State(s) in (\"\")"=w310) -> ("States Out"=w309:string)  [unwired: 13 in]
          }
          frame "---------- Process ----------" {
            # "Template Separator\n(You can make a copy of, or modify, this frame)"
            n104 = call <vilib>:"Add State(s) to Queue__jki_lib_state_machine.vi"("State(s) in (\"\")"=w315) -> ("States Out"=w314:string)  [unwired: 14 in]
          }
          frame "Process: Sync" {
            n105 = Unbundle By Name(w323) -> ("Self Reference"=w316:refnum<class "RemoteControl.lvclass">)
            n106 = call <vilib>:"WaitOnProcessSync.vi"("error in (no error)"=w319, "SMO"=w316) -> ("error out"=w318:errorcluster, "Don't run?"=w322:bool)  [unwired: 7 in, 1 out]
            n107 = Select(t="Data: Cleanup\nEvents: Unregister\nExit", s=w322, f="") -> (s? t:f=w317:string)
            n108 = call <vilib>:"Add State(s) to Queue__jki_lib_state_machine.vi"("State(s) in Front (\"\")"=w317, "State(s) in (\"\")"=w326) -> ("States Out"=w325:string)  [unwired: 13 in]
          }
          frame "Process: SelfTerminate" {
            n109 = Unbundle By Name(w331) -> ("Self Reference"=w330:refnum<class "RemoteControl.lvclass">)
            n110 = call <vilib>:"SelfTerminate.vi"("error in (no error)"=w328, "SMO in"=w330) -> ("error out"=w327:errorcluster, "SMO out"=w329:refnum<class "RemoteControl.lvclass">)  [unwired: 8 in]
            n111 = Bundle By Name(cluster=w331, "Self Reference"=w329) -> (w332:T8)
            n112 = call <vilib>:"Add State(s) to Queue__jki_lib_state_machine.vi"("State(s) in (\"\")"=w335) -> ("States Out"=w334:string)  [unwired: 14 in]
          }
          frame "---------- Events ----------" {
            # "Template Separator\n(You can make a copy of, or modify, this frame)"
            n113 = call <vilib>:"Add State(s) to Queue__jki_lib_state_machine.vi"("State(s) in (\"\")"=w340) -> ("States Out"=w339:string)  [unwired: 14 in]
          }
          frame "Events: Register" {
            (unwired) refnum<user-event>[] [] items=["unknown", "Created", "Started", "Stopped"]  # Server State
            (unwired) refnum<user-event>[] []  # Message From Server
            # "Expand to add\nmore events"
            n114 = Unbundle By Name(w357) -> ("Self Reference"=w348:refnum<class "RemoteControl.lvclass">)
            n115 = call <vilib>:"GetProtectedEvents.vi"("SMO"=w348) -> ("error out"=w351:errorcluster, "SMO Protected Events"=w355:T10, "SMO out"=w347:refnum<class "RemoteControl.lvclass">)  [unwired: 8 in]
            n116 = call "RemoteControl.GetPrivateEvents.vi"("RemoteControl"=w347) -> ("error out"=w349:errorcluster, "RC Private Events"=w350:T11, "RemoteControl out"=w343:refnum<class "RemoteControl.lvclass">)  [unwired: 8 in]
            n117 = call "RemoteControl.GetPublicEvents.vi"("RemoteControl"=w343) -> ("error out"=w342:errorcluster, "RC Public Events"=w346:T12, "RemoteControl out"=w345:refnum<class "RemoteControl.lvclass">)  [unwired: 8 in]
            n118 = Unbundle(w346) -> ()  [unwired: 1 out]
            n119 = call <vilib>:"GetPublicEvents.vi"("SMO"=w345) -> ("error out"=w341:errorcluster, "Public Events"=w344:T13)  [unwired: 8 in, 1 out]
            n120 = Unbundle By Name(w344) -> ()  [unwired: 1 out]
            n121 = register-events(w355, w350) -> (reference out=w356:refnum<event-registration>, error out=w352:errorcluster)  [unwired: 2 in]
            n122 = Merge Errors(w341, w342, w349, w354, w352, w351) -> (w353:errorcluster)
            n123 = call <vilib>:"Add State(s) to Queue__jki_lib_state_machine.vi"("State(s) in (\"\")"=w359) -> ("States Out"=w358:string)  [unwired: 14 in]
          }
          frame "Events: Unregister" {
            n124 = Unregister For Events(event registration refnum=w362, error in=w361) -> (error out=w360:errorcluster)
            n125 = call <vilib>:"Clear Errors.vi"("error in (no error)"=w360) -> ()  [unwired: 5 in, 2 out]
            n126 = call <vilib>:"Add State(s) to Queue__jki_lib_state_machine.vi"("State(s) in (\"\")"=w365) -> ("States Out"=w364:string)  [unwired: 14 in]
          }
          frame "---------- RC ----------" {
            # "Template Separator\n(You can make a copy of, or modify, this frame)"
            n127 = call <vilib>:"Add State(s) to Queue__jki_lib_state_machine.vi"("State(s) in (\"\")"=w370) -> ("States Out"=w369:string)  [unwired: 14 in]
          }
          frame "RC: Open Context" {
            n128 = Unbundle By Name(w372) -> ("Self Reference"=w374:refnum<class "RemoteControl.lvclass">)
            n129 = call-dynamic "Open Context.vi"("error in (no error)"=w375, "RemoteControl in"=w374) -> ("error out"=w376:errorcluster, "RemoteControl out"=w371:refnum<class "RemoteControl.lvclass">)  [unwired: 8 in]
            n130 = Bundle By Name(cluster=w372, "Self Reference"=w371) -> (w373:T8)
            n131 = call <vilib>:"Add State(s) to Queue__jki_lib_state_machine.vi"("State(s) in (\"\")"=w379) -> ("States Out"=w378:string)  [unwired: 14 in]
          }
          frame "RC: Send Message to Owner" {
            # "Send Message to Owner to be processed\n(Send a message to the instrument to be processed)"
            n132 = Unbundle By Name(w388) -> ("Self Reference"=w386:refnum<class "RemoteControl.lvclass">, "Message"=w380:T1)
            n133 = call "Time Message Events.vi"("error in (no error)"=w382, "Debug Mode"=w383, "Message in"=w380) -> ("error out"=w381:errorcluster, "Message out"=w384:T1)  [unwired: 6 in, 1 out]
            n134 = Bundle("Message out"=w384) -> (w385:cluster{"Message out":T1})  [unwired: 1 in]
            n135 = call "RemoteControl.SendMessageFromProcess.vi"("error in (no error)"=w381, "SendMessageFromProcess"=w385, "RemoteControl"=w386) -> ("error out"=w387:errorcluster)  [unwired: 7 in, 1 out]
            n136 = call <vilib>:"Add State(s) to Queue__jki_lib_state_machine.vi"("State(s) in (\"\")"=w391) -> ("States Out"=w390:string)  [unwired: 14 in]
          }
          frame "RC: Get Connections" {
            # "Here listen for new connections and then stop after timeout or if there's a new connection"
            n137 = Unbundle By Name(w393) -> ("Self Reference"=w398:refnum<class "RemoteControl.lvclass">)
            n138 = call-dynamic "Get Connections.vi"("error in (no error)"=w397, "RemoteControl in"=w398) -> ("error out"=w396:errorcluster, "Numeric"=w395:i32, "RemoteControl out"=w392:refnum<class "RemoteControl.lvclass">)  [unwired: 7 in]
            n139 = Bundle By Name(cluster=w393, "Self Reference"=w392) -> (w394:T8)
            n140 = case shown="1" w395 {
              tunnel: ["" ("State(s) in Front (\"\")") "RC: Read Messages" ("State(s) in Front (\"\")") "RC: Close Connection" ("State(s) in Front (\"\")")] -> w399
              frame 0 {
              }
              frame 1 {
              }
              frame Default {
              }
            }
            n141 = call <vilib>:"Add State(s) to Queue__jki_lib_state_machine.vi"("State(s) in Front (\"\")"=w399, "State(s) in (\"\")"=w402) -> ("States Out"=w401:string)  [unwired: 13 in]
          }
          frame "RC: Read Messages" {
            # "Read Message over, eg TCP"
            # "If command is empty do not Send Message"
            n142 = Unbundle By Name(w408) -> ("Message"=w411:T1, "Self Reference"=w417:refnum<class "RemoteControl.lvclass">)
            n143 = call-dynamic "Read Message.vi"("timeout in ms (100)"="timeout in ms (100)", "error in (no error)"=w418, "RemoteControl in"=w417) -> ("error out"=w410:errorcluster, "Data"=w413:variant, "Command"=w414:string, "Message ID"=w412:i32)  [unwired: 4 in, 1 out]
            n144 = case shown="Default" w414 {
              selector: w414 -> [w432 _]
              tunnel: ["RC: Send Message to Owner" ("State(s) in Front (\"\")") "" ("State(s) in Front (\"\")")] -> w416
              tunnel: w413 -> [w431 _]
              tunnel: w412 -> [w430 _]
              tunnel: w411 -> [w429 _]
              tunnel: w410 -> [w428 w434]
              tunnel: [w427 w434] -> w409
              tunnel: w408 -> [w426 w435]
              tunnel: [w425 w435] -> w407
              tunnel: w406 -> [w424 _]
              frame Default {
                n145 = Bundle By Name(cluster=w429, "Command"=w432, "Data"=w431, "Message ID"=w430) -> (w422:T1)
                "Message from Remote" <- w422
                n146 = call "Time Message Events.vi"("error in (no error)"=w428, "Debug Mode"=w424, "Message in"=w422) -> ("error out"=w427:errorcluster, "Message out"=w433:T1)  [unwired: 6 in, 1 out]
                n147 = Bundle By Name(cluster=w426, "Message"=w433) -> (w425:T8)
              }
              frame "" {
              }
            }
            n148 = call <vilib>:"Add State(s) to Queue__jki_lib_state_machine.vi"("State(s) in Front (\"\")"=w416, "State(s) in (\"\")"=w421) -> ("States Out"=w420:string)  [unwired: 13 in]
          }
          frame "RC: Write Messages" {
            # "send Message over, eg. TCP"
            n149 = Unbundle By Name(w445) -> ("Self Reference"=w447:refnum<class "RemoteControl.lvclass">, "Message"=w443:T1)
            n150 = call "Time Message Events.vi"("error in (no error)"=w442, "Debug Mode"=w444, "Message in"=w443) -> ("error out"=w441:errorcluster, "Message out"=w440:T1)  [unwired: 6 in, 1 out]
            n151 = Unbundle By Name(w440) -> ("Command"=w439:string, "Data"=w438:variant, "Message ID"=w437:i32)
            n152 = call-dynamic "Send Message.vi"("Message ID"=w437, "error in (no error)"=w441, "Data"=w438, "Command"=w439, "RemoteControl in"=w447) -> ("error out"=w446:errorcluster)  [unwired: 5 in, 1 out]
            n153 = call <vilib>:"Add State(s) to Queue__jki_lib_state_machine.vi"("State(s) in (\"\")"=w450) -> ("States Out"=w449:string)  [unwired: 14 in]
          }
          frame "RC: Close Connection" {
            # "Closes open server connections"
            # "call this on error 66, etc (when connection\ndrops). check these in error handler"
            n154 = Unbundle By Name(w455) -> ("Self Reference"=w456:refnum<class "RemoteControl.lvclass">)
            n155 = call-dynamic "Close Connection.vi"("error in (no error)"=w452, "RemoteControl in"=w456) -> ("error out"=w451:errorcluster, "RemoteControl out"=w453:refnum<class "RemoteControl.lvclass">)  [unwired: 8 in]
            n156 = Bundle By Name(cluster=w455, "Server"=w453) -> (w454:T8)
            n157 = call <vilib>:"Add State(s) to Queue__jki_lib_state_machine.vi"("State(s) in (\"\")"=w459) -> ("States Out"=w458:string)  [unwired: 14 in]
          }
          frame "RC: Stop Listener" {
            # "Stop Asynchronous Listener \n(You can make a copy of, or modify, this frame)"
            n158 = Unbundle By Name(w463) -> ("Self Reference"=w462:refnum<class "RemoteControl.lvclass">)
            n159 = call-dynamic "Connection Monitor - Stop.vi"("error in (no error)"=w461, "RemoteControl in"=w462) -> ("error out"=w460:errorcluster)  [unwired: 8 in, 1 out]
            n160 = call <vilib>:"Add State(s) to Queue__jki_lib_state_machine.vi"("State(s) in (\"\")"=w466) -> ("States Out"=w465:string)  [unwired: 14 in]
          }
          frame "RC: Open Client Connection" {
            n161 = Unbundle By Name(w468) -> ("Self Reference"=w472:refnum<class "RemoteControl.lvclass">)
            n162 = call-dynamic "Open Client Connection.vi"("error in (no error)"=w471, "RemoteControl in"=w472) -> ("error out"=w470:errorcluster, "RemoteControl out"=w469:refnum<class "RemoteControl.lvclass">)  [unwired: 8 in]
            n163 = Bundle By Name(cluster=w468, "Self Reference"=w469) -> (w467:T8)
            n164 = call <vilib>:"Add State(s) to Queue__jki_lib_state_machine.vi"("State(s) in (\"\")"=w475) -> ("States Out"=w474:string)  [unwired: 14 in]
          }
          frame "RC: Open Server Connection" {
            n165 = Unbundle By Name(w483) -> ("Self Reference"=w481:refnum<class "RemoteControl.lvclass">, "Configure.address"=w477:string, "Configure.Port"=w476:u16)
            n166 = call-dynamic "Build Endpoint.vi"("error in (no error)"=w478, "Port"=w476, "Address"=w477, "RemoteControl in"=w481) -> ("error out"=w479:errorcluster, "RemoteControl out"=w480:refnum<class "RemoteControl.lvclass">)  [unwired: 6 in]
            n167 = call-dynamic "Open Server Connection.vi"("error in (no error)"=w479, "RemoteControl in"=w480) -> ("error out"=w485:errorcluster, "RemoteControl out"=w482:refnum<class "RemoteControl.lvclass">)  [unwired: 8 in]
            n168 = Bundle By Name(cluster=w483, "Self Reference"=w482) -> (w484:T8)
            n169 = call <vilib>:"Add State(s) to Queue__jki_lib_state_machine.vi"("State(s) in (\"\")"=w488) -> ("States Out"=w487:string)  [unwired: 14 in]
          }
        }
      }
    }
    frame Error {
    }
  }
  n170 = call-parent "Process.vi"("error in"=w2, "LevyLab"=w1) -> ("error out"=w5:errorcluster, "LevyLab out"=→"RemoteControl out":refnum<class "RemoteControl.lvclass">)  [unwired: 8 in]
  n171 = call-dynamic "Connection Monitor - Loop.vi"("error in (no error)"=w2, "RemoteControl in"=w1) -> ("error out"=w3:errorcluster)  [unwired: 8 in, 1 out]
  n172 = Merge Errors(w3, w5) -> (w4:errorcluster)
  n173 = Merge Errors(w4, w9) -> (→"error out":errorcluster)
